vi "Write License to File.vi"(8 "error in (no error)":errorcluster caption="错误输入（无错误）", 11 "Input License":string) -> (0 "error out":errorcluster caption="错误输出")   [LabVIEW 2011]
doc: "将用户输入许可证号码写入文件"
uses:
  <vilib>/Utility/config.llb/Write Key (String).vi
  <vilib>/Utility/config.llb/NI_LVConfig.lvlib
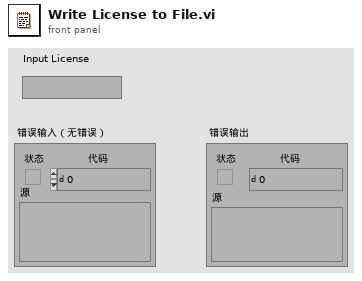
[diagram p1: front panel]
types:
  T1 = enum32{"invalid app kind", "Development System", "Run Time System", "Student Edition", "Embedded LabVIEW", "Evaluation", "Custom"}
  T2 = typedef "NI_LVConfig.lvlib/Config Data RefNum.ctl" = refnum<k1>
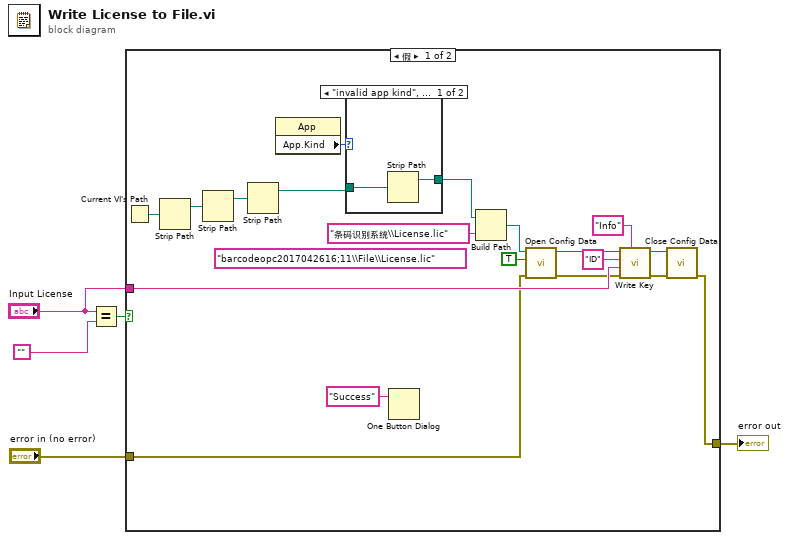
[diagram p0: block diagram]
diagram:
  n1 = Equal?(x="Input License", y="") -> (x = y?=w5:bool)
  n2 = case shown="假" w5 {
    tunnel: "Input License" -> [w21 _]
    tunnel: [w10 w28] -> w2
    tunnel: "error in (no error)" -> [w9 w28]
    frame False {
      (unwired) "barcodeopc2017042616;11\\File\\License.lic" ("名称或相对路径")
      n3 = Current VI's Path() -> (path=w19:path)
      n4 = Strip Path(path=w19) -> (stripped path=w18:path)  [unwired: 1 out]
      n5 = Strip Path(path=w18) -> (stripped path=w14:path)  [unwired: 1 out]
      n6 = Strip Path(path=w14) -> (stripped path=w7:path)  [unwired: 1 out]
      n7 = property class="App"() -> ("App.Kind"=w15:T1)  [unwired: 2 in, 2 out]
      n8 = case shown="\"invalid app kind\", 默认" w15 {
        tunnel: w7 -> [w26 w27]
        tunnel: [w25 w27] -> w8
        frame "invalid app kind", Default {
          n9 = Strip Path(path=w26) -> (stripped path=w25:path)  [unwired: 1 out]
        }
        frame "Development System" {
        }
      }
      n10 = One Button Dialog(message="Success" ("消息")) -> ()  [unwired: 1 in, 1 out]
      n11 = Build Path(base path=w8, name or relative path="条码识别系统\\License.lic" ("名称或相对路径")) -> (appended path=w16:path)
      n12 = call <vilib>:"Open Config Data.vi"("error in (no error)"=w9, "create file if necessary (T)"=TRUE, "configuration file path"=w16) -> ("error out"=w12:errorcluster, "refnum"=w24:T2)  [unwired: 6 in, 1 out]
      n13 = call-poly <vilib>:"Write Key.vi"("section"="Info", "error in (no error)"=w12, "value"=w21, "key"="ID", "refnum"=w24) -> ("error out"=w11:errorcluster, "refnum out"=w20:T2)  [unwired: 4 in, 1 out]
      n14 = call <vilib>:"Close Config Data.vi"("error in (no error)"=w11, "refnum"=w20) -> ("error out"=w10:errorcluster)  [unwired: 8 in, 1 out]
    }
    frame True {
    }
  }
  "error out" <- w2
